vi "e1039_Magnet_PS_Control.vi"(10 "Comms Layer":T1=enum."ISOBus - RS-232", 11 "Serial Port":refnum<visa-resource-name>="COM6") -> (3 "Output Current (A)":dbl format="%.2g")   [LabVIEW 2019]
uses:
  Mercury iXX Modules/Public/Controls/Comms Transport Layer.ctl
  Mercury iXX Modules/Public/Controls/ISOBus Address.ctl
  Mercury iXX Modules/Public/Controls/Serial Settings.ctl
  Mercury iXX Modules/Public/Libraries/Magnet/Controls/Switch Heater.ctl
  Mercury iXX Modules/Public/Libraries/Magnet/Controls/PSU Actions.ctl
  Mercury iXX Modules/Public/Libraries/System/Open/Open System.vi
  Mercury iXX Modules/Public/Libraries/System/Read/Catalogue (Read).vi
  Global 2.vi
  Mercury iXX Modules/Public/Libraries/Magnet/Open/Open Magnet Device.vi
  Mercury iXX Modules/Public/Libraries/Magnet/Signals/Read/Persistant Current (Read).vi
  Mercury iXX Modules/Public/Libraries/Magnet/Signals/Read/Current (Read).vi
  Mercury iXX Modules/Public/Libraries/Magnet/Signals/Read/Voltage (Read).vi
  Mercury iXX Modules/Public/Libraries/Magnet/Signals/Read/Switch Heater Status (Read).vi
  Mercury iXX Modules/Public/Libraries/Magnet/Signals/Set/Switch Heater No Check (Set).vi
  Mercury iXX Modules/Public/Libraries/Magnet/Configuration/Set/PSU Action Status (Set).vi
  Mercury iXX Modules/Public/Libraries/Magnet/Signals/Set/Target Current (Set).vi
  Mercury iXX Modules/Public/Libraries/Magnet/Signals/Set/Target Current Rate (Set).vi
  Mercury iXX Modules/Public/Libraries/Magnet/Configuration/Read/PSU Action Status (Read).vi
  Mercury iXX Modules/Public/Libraries/Level Meter/Signals/Read/Probe Level Helium (Read).vi
  Mercury iXX Modules/Public/Libraries/Level Meter/Signals/Read/Probe Level Nitrogen (Read).vi
  Mercury iXX Modules/Mercury iXX.lvlib
  Mercury iXX Modules/Public/Libraries/Magnet.lvlib
  Mercury iXX Modules/Public/Libraries/System.lvlib
  Mercury iXX Modules/Public/Libraries/Level Meter.lvlib
panel:
  in  "Stop Button":bool
  out "Shim Relay Message":string
  out "Shim Relay Status":bool
  in  "Shim Relay SN":string="AB0NXJH7"
  out "Shim2Light":bool
  in  "Shim 2":bool
  out "Shim1Light":bool
  in  "Shim 1":bool
  in  "OK Button":bool
  in  "x":dbl=14.889566783098592 format="%#_13g"
  in  "Current NMR Central Frequency:":dbl
  in  "y":dbl=20.0
  out "SAFETY TIMEOUT":u8(slide) scale=0.0..60.0
  in  "safemode":bool=TRUE
  out "Numeric":dbl
  in  "Help Button":bool
  out "help":string="To ramp the current above 74.8 A, or faster than 2 A/min (for I<40A), 1 A/min (for 40A<I<63A) or 0.5 A/min (for I>63A), please enter the correct password.\n\nBaseline Mode: Toggle on to ramp the magnet to 1 A below the set point for the purposes of taking a baseline. Toggle off to ramp back to the set point. If the switch heater is off, it will be turned on when this button is pressed.\n\nSafety Mode: While toggled on, switch heater will automatically turn off after 20 minutes of inactivity. Enter password to change timeout duration."
  in  "Special Functions":bool
  out "Baselinetext":string
  in  "Target Species:":dbl(ring)=42.576 items=["Proton"=42.576, "Deuteron"=6.536]
  out "Heater Status 2":u8(slide) scale=0.0..60.0
  in  "Baseline Mode":bool
  out "Heater Status":u8(slide) scale=0.0..60.0
  out "String":string
  in  "Target Frequency (MHz):":dbl max=213.8870019787944
  in  "Target Field (T):":dbl max=5.02365186909983 format="%#_5g"
  in  "Axis Group":string(combo)="GRPZ"
  in  "Target Current":dbl max=74.8 format="%#_5g"
  out "concatenated string 2":string
  out "Nitrogen Fill Level":dbl(slide) scale=0.0..100.0
  out "concatenated string":string
  out "Helium Fill Level":dbl(slide) scale=0.0..100.0
  in  "stop":bool
  in  "controlslock":bool
  out "Zerolight":bool
  out "Setlight":bool
  out "Holdlight":bool
  out "Persistent Current (A)":dbl format="%.2g"
  in  "PASSWORD:":string
  out "Heater Indicator 3":bool
  in  "Switch Heater":bool
  in  "Ramp Rate (A/min)":dbl=0.5 min=0.0 max=2.0 format="%_6g"
  out "Target Current (A):":cluster{dbl, dbl}(knob)={0.0, 68.56622626412835} scale=0.0..120.0 scale format="%#_5g"
  in  "To Zero":bool
  in  "To Set":bool
  in  "Hold":bool
  out "Waveform Chart":cluster{"[0]":dbl, "[1]":dbl}(graph)
  out "Output Voltage (V)":dbl format="%.3g"
  out "Connected?":bool
  out "String 2":string
  # "Fermilab e1039 Magnet Control"
  # "For Drift Calibration:"
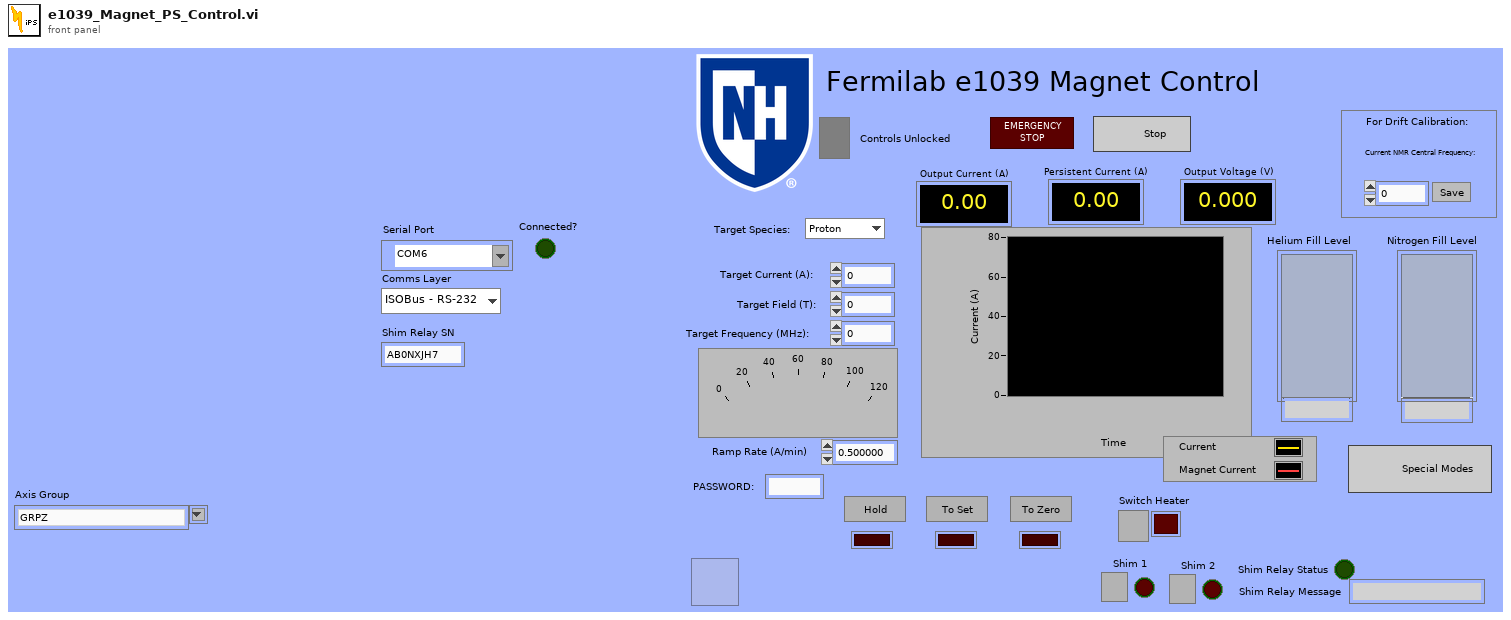
[diagram p1: front panel]
types:
  T1 = typedef "Mercury iXX.lvlib/Comms Transport Layer.ctl" = enum16{"Ethernet TCP/IP", "USB", "ISOBus - RS-232", "GPIB"}
  T2 = typedef "Mercury iXX.lvlib/Serial Settings.ctl" = cluster{"Baud Rate":u32, "Parity":u16, "Data Bits":u16, "Stop Bits":u16, "Flow Control":u16}
  T3 = typedef "Mercury iXX.lvlib/ISOBus Address.ctl" = i32
  T4 = typedef "Mercury iXX.lvlib/Mercury Reference.ctl" = cluster{"Comms":refnum<visa-resource-name>, "Device ID":string[], "Comms Layer":T1, "Command":string, "Query reference":T5}
  T5 = typedef "Mercury iXX.lvlib/Query Dynamic Reference.ctl" = refnum<vi>
  T6 = enum8{"Enabled", "Disabled", "Disabled and Grayed Out"}
  T7 = typedef "Mercury iXX.lvlib/Magnet.lvlib/PSU Actions.ctl" = string
  T8 = typedef "Mercury iXX.lvlib/Magnet.lvlib/Switch Heater.ctl" = string
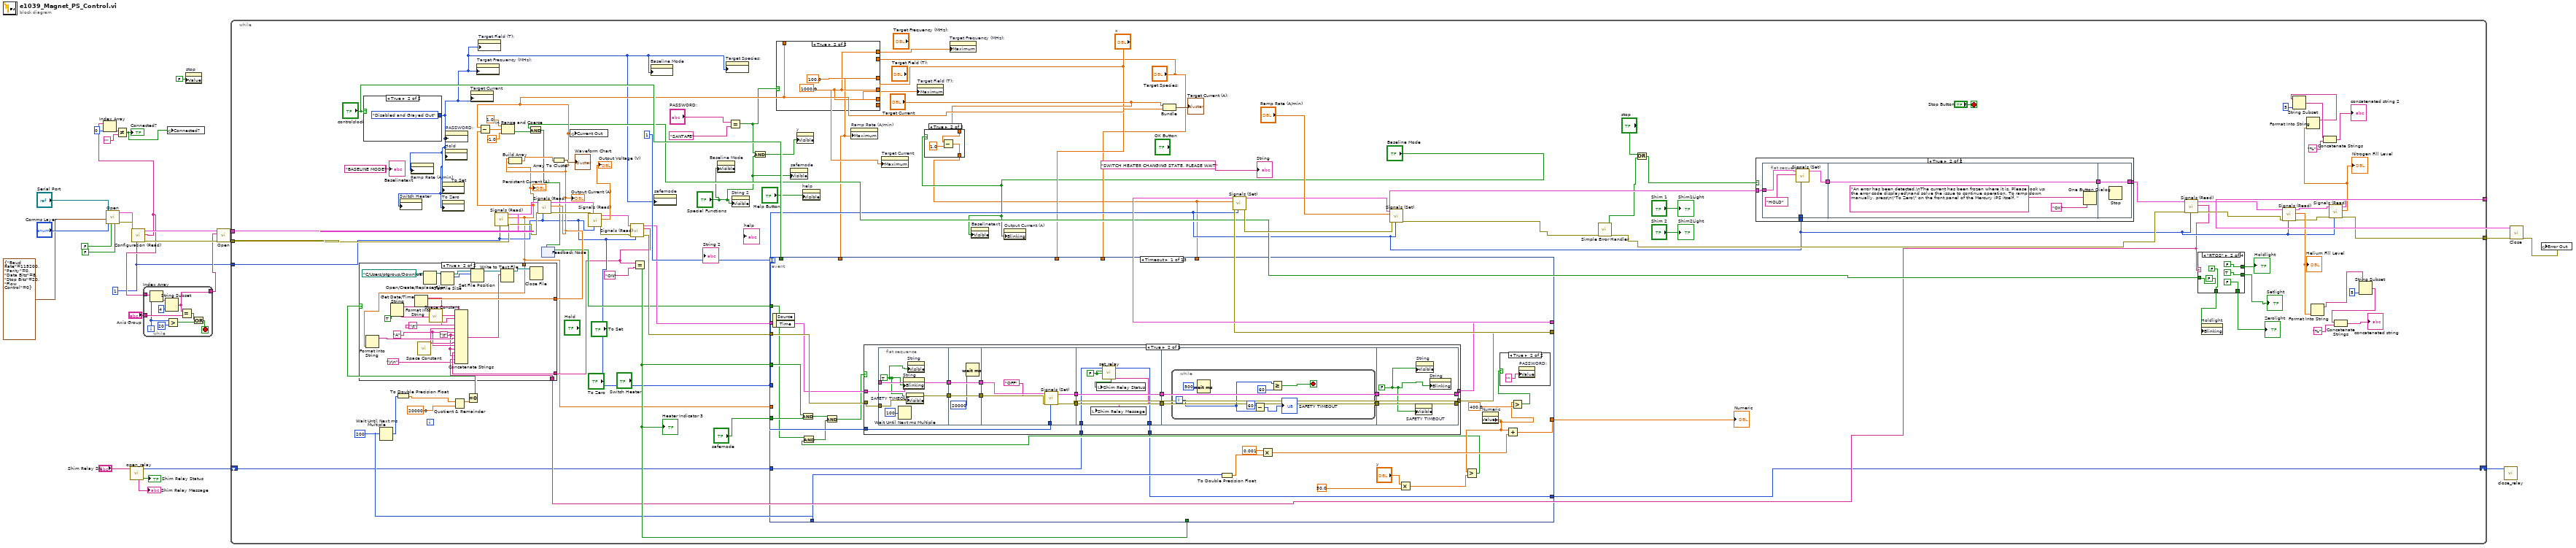
[diagram p0: block diagram]
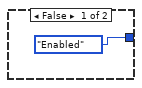
[diagram p3: hidden frame]
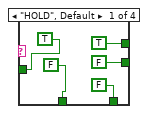
[diagram p4: hidden frame]
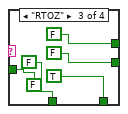
[diagram p5: hidden frame]
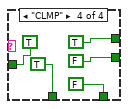
[diagram p6: hidden frame]
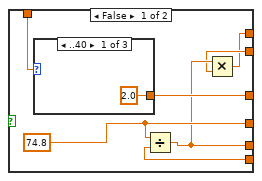
[diagram p9: hidden frame]
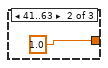
[diagram p10: hidden frame]
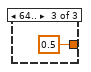
[diagram p11: hidden frame]
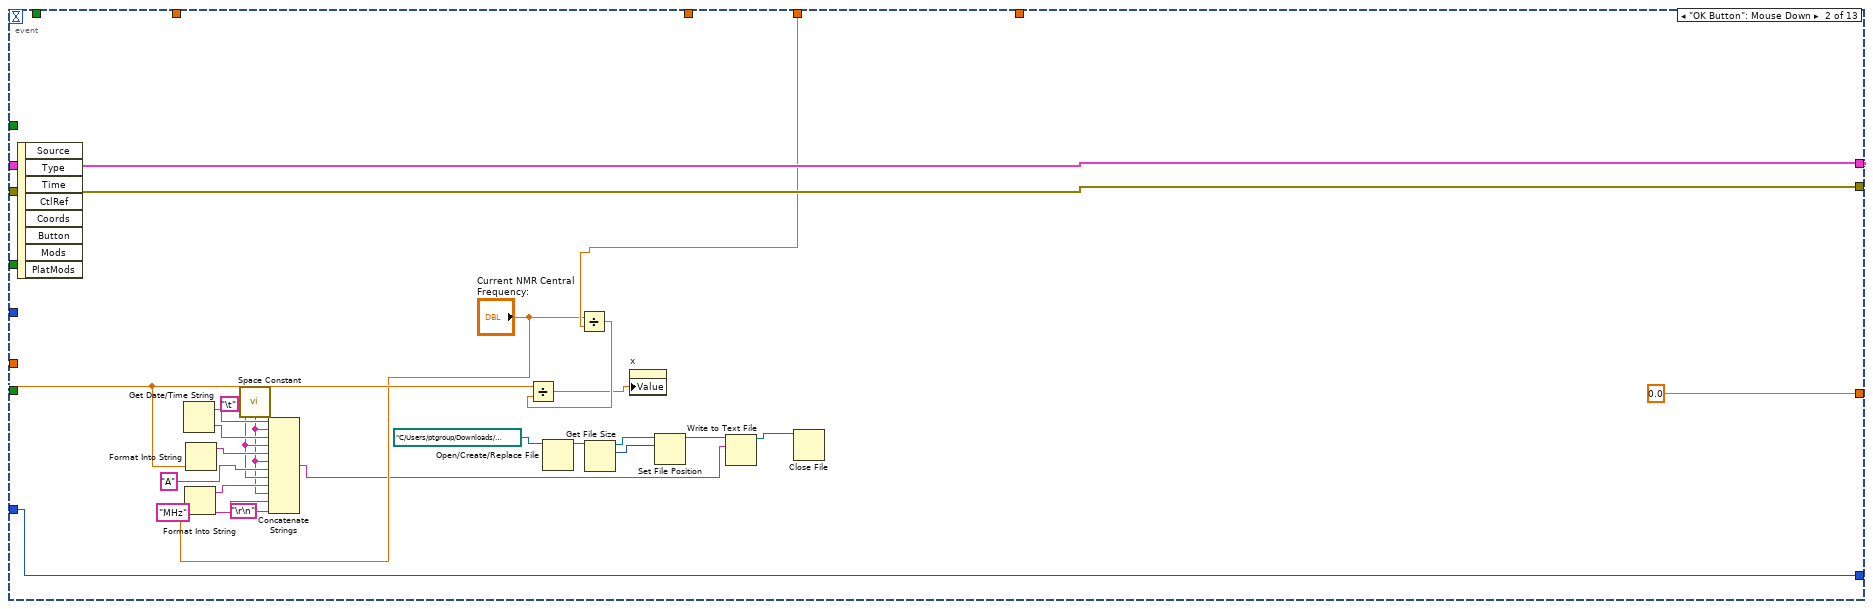
[diagram p14: hidden frame]
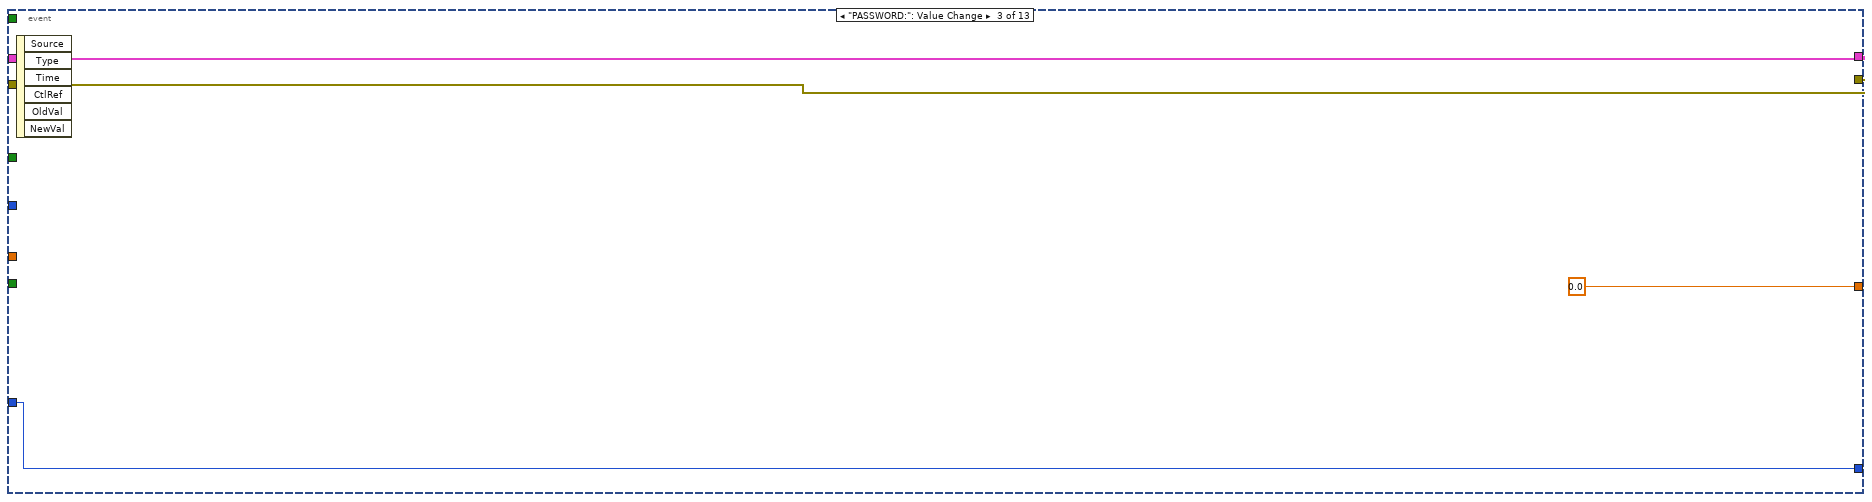
[diagram p15: hidden frame]
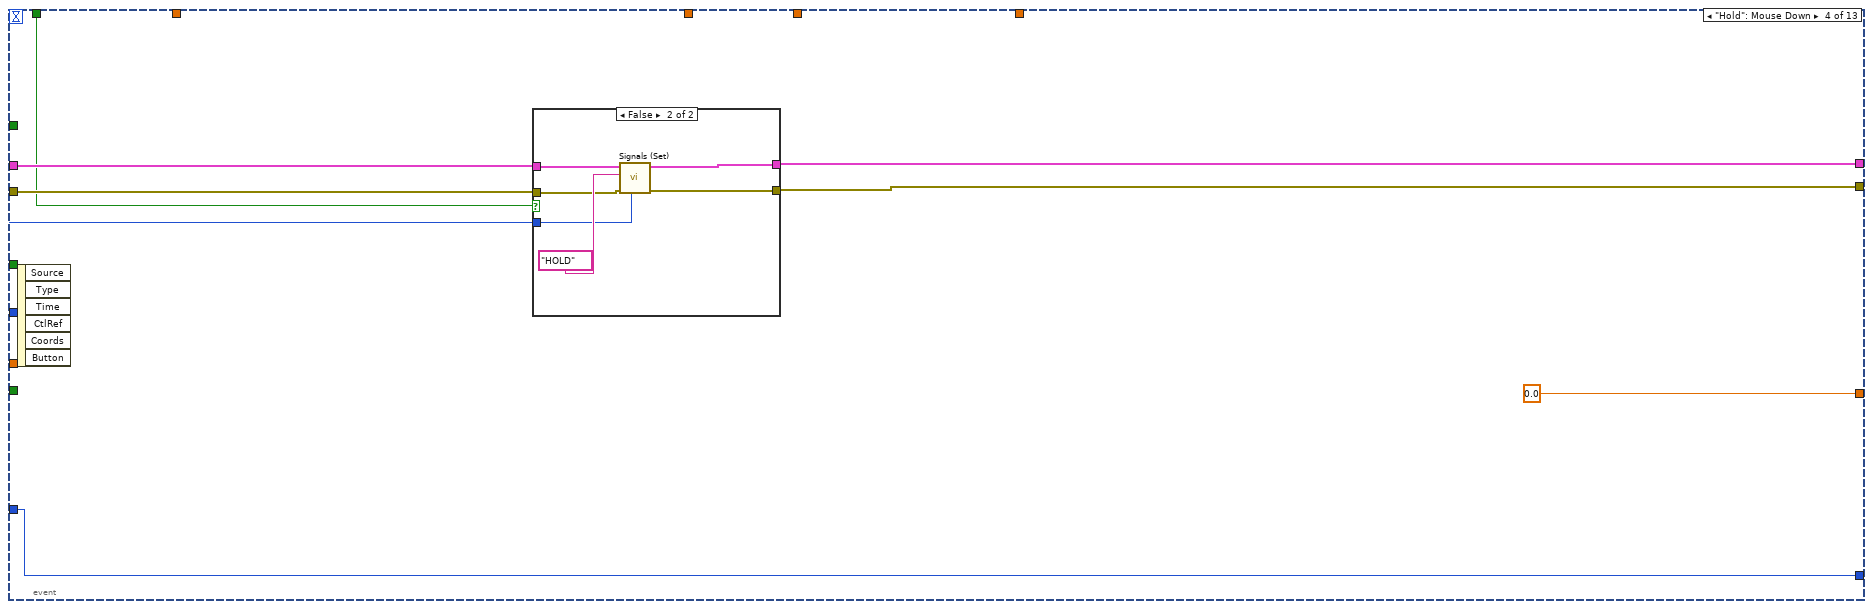
[diagram p16: hidden frame]
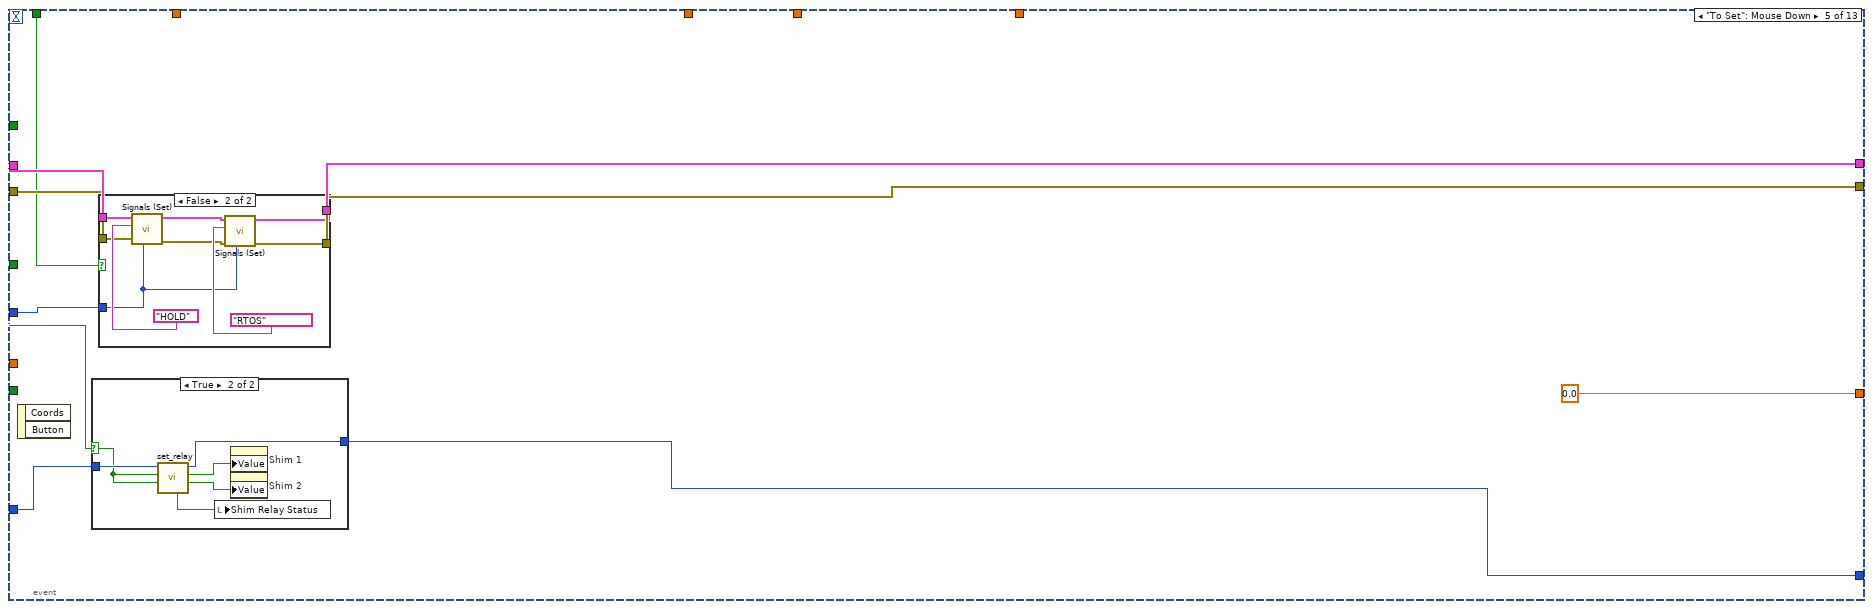
[diagram p18: hidden frame]
diagram:
  w7 = T3 1 ("ISOBUS address")
  n1 = call-poly "Open.vi"("Clear Previous Connections (False)"=FALSE, "ID Query (True)"=FALSE, "Serial Configuration"=T2 {"Baud Rate"=115200, "Parity"=0, "Data Bits"=8, "Stop Bits"=20, "Flow Control"=0}, "Comms Layer"="Comms Layer", "VISA resource name"="Serial Port") -> ("error out"=w21:errorcluster, "Mercury Reference Out"=w27:T4)  [unwired: 2 in, 3 out]
  n2 = call "open_relay.vi"("serial_number"="Shim Relay SN") -> ("status"=→"Shim Relay Status":bool, "Handle"=w2:u64, "message"=→"Shim Relay Message":string)  [unwired: 7 in, 1 out]
  n3 = call-poly "Configuration (Read).vi"("ISOBUS address"=w7, "error in"=w21, "Mercury Reference In"=w27) -> ("error out"=w20:errorcluster, "Devices"=w9:string[], "Mercury Reference Out"=w23:T4)  [unwired: 5 in, 1 out]
  n4 = Index Array(array=w9, index=0) -> (element=w24:string)
  n5 = Not Equal?(x=w24, y="") -> (x != y?=w6:bool)
  "Connected?" <- w6
  n6 = while {
    tunnel: w9 -> [w38]
    tunnel: [w29] -> w8
    tunnel: "Axis Group" -> [w35]
    i -> [w33]
    stop <- w32 stop-if-true
    n7 = Index Array(array=w38, index=w33) -> (element=w36:string)
    n8 = String Subset(string=w36, length (rest)=4 ("length (rest)")) -> (substring=w29:string)  [unwired: 1 out]
    n9 = Greater?(x=w33, y=20) -> (0:w31:bool)
    n10 = Equal?(x=w29, y=w35) -> (x = y?=w30:bool)
    n11 = Or(x=w30, y=w31) -> (x .or. y?=w32:bool)
  }
  n12 = global write "Global 2.vi" "Connected?"(w6) -> ()
  n13 = property on="stop" class="Bool (strict)"("Value"=FALSE ("stop")) -> ()  [unwired: 2 in, 2 out]
  n14 = call-poly "Open.vi"("error in (no error)"=w20, "Device Identifier"=w8, "Mercury Reference In"=w23) -> ("error out"=w19:errorcluster, "Mercury Reference Out"=w22:T4)  [unwired: 7 in]
  n15 = while {
    tunnel: w22 -> [w113]
    tunnel: w19 -> [w115]
    tunnel: [w86] -> w17
    tunnel: [w85] -> w16
    tunnel: w7 -> [w65]
    shift-right: [w40] -> w1
    shift-left: w2 -> [w41]
    stop <- "Stop Button" stop-if-true
    (unwired) "BASELINE MODE" ("Baselinetext")
    w51 = u32 200 ("millisecond multiple")
    n16 = case shown="True" "controlslock" {
      tunnel: [T6."Enabled" ("Disabled") T6."Disabled and Grayed Out" ("Disabled")] -> w45
      frame False {
      }
      frame True {
      }
    }
    n17 = Wait Until Next ms Multiple(millisecond multiple=w51) -> (millisecond timer value=w110:u32)
    n18 = To Double Precision Float(number=w110) -> (double precision float=w107:dbl)
    n19 = property on="Switch Heater" class="Bool (strict)"("DisabledEnum"=w45) -> ()  [unwired: 2 in, 2 out]
    n20 = property on="Ramp Rate (A/min)" class="DigNum (strict)"("DisabledEnum"=w45) -> ()  [unwired: 2 in, 2 out]
    n21 = property on="To Set" class="Bool"("DisabledEnum"=w45) -> ()  [unwired: 2 in, 2 out]
    n22 = property on="To Zero" class="Bool"("DisabledEnum"=w45) -> ()  [unwired: 2 in, 2 out]
    n23 = property on="Hold" class="Bool"("DisabledEnum"=w45) -> ()  [unwired: 2 in, 2 out]
    n24 = property on="PASSWORD:" class="Str"("DisabledEnum"=w45) -> ()  [unwired: 2 in, 2 out]
    n25 = Quotient & Remainder(x=w107, y=20000.0) -> (x-y*floor(x/y)=w108:dbl)  [unwired: 1 out]
    n26 = Equal To 0?(x=w108) -> (x = 0?=w109:bool)
    n27 = property on="Target Current" class="DigNum (strict)"("DisabledEnum"=w45) -> ()  [unwired: 2 in, 2 out]
    n28 = property on="Target Frequency (MHz):" class="DigNum (strict)"("DisabledEnum"=w45) -> ()  [unwired: 2 in, 2 out]
    n29 = property on="Target Field (T):" class="DigNum (strict)"("DisabledEnum"=w45) -> ()  [unwired: 2 in, 2 out]
    n30 = call-poly "Signals (Read).vi"("ISOBUS address"=w65, "error in"=w115, "Mercury Reference In"=w113) -> ("error out"=w114:errorcluster, "Persistant Current"=w46:dbl, "Mercury Reference Out"=w112:T4)  [unwired: 4 in, 2 out]
    "Persistent Current (A)" <- w46
    n31 = call-poly "Signals (Read).vi"("ISOBUS address"=w65, "error in"=w114, "Mercury Reference In"=w112) -> ("error out"=w124:errorcluster, "Current"=w72:dbl, "Mercury Reference Out"=w133:T4)  [unwired: 4 in, 2 out]
    "Output Current (A)" <- w72
    n32 = Subtract(x=w72, y=w46) -> (x-y=w106:dbl)
    n33 = In Range and Coerce(upper limit=1.0, x=w106, lower limit=-1.0) -> (In Range?=w69:bool)  [unwired: 1 out]
    n34 = Build Array(w72, w46) -> (w80:dbl[])
    n35 = feedback #1() -> (w66:bool)  [unwired: 1 in]
    n36 = Array To Cluster(array=w80) -> (cluster=→"Waveform Chart":cluster{"[0]":dbl, "[1]":dbl})
    n37 = global write "Global 2.vi" "Current Out"(w72) -> ()
    n38 = call-poly "Signals (Read).vi"("ISOBUS address"=w65, "error in"=w124, "Mercury Reference In"=w133) -> ("error out"=w123:errorcluster, "Voltage"=→"Output Voltage (V)":dbl, "Mercury Reference Out"=w127:T4)  [unwired: 4 in, 2 out]
    n39 = call-poly "Signals (Read).vi"("ISOBUS address"=w65, "error in"=w123, "Mercury Reference In"=w127) -> ("error out"=w121:errorcluster, "Switch Heater Status"=w56:string, "Mercury Reference Out"=w126:T4)  [unwired: 5 in, 1 out]
    n40 = Equal?(x=w56, y="ON") -> (x = y?=w97:bool)
    "Heater Indicator 3" <- w97
    n41 = property on="Baseline Mode" class="Bool (strict)"("DisabledEnum"=w45) -> ()  [unwired: 2 in, 2 out]
    n42 = property on="safemode" class="Bool (strict)"("DisabledEnum"=w45) -> ()  [unwired: 2 in, 2 out]
    n43 = property on="Baseline Mode" class="Bool (strict)"("Visible"="Special Functions") -> ()  [unwired: 2 in, 2 out]
    n44 = property on="Target Species:" class="Ring (strict)"("DisabledEnum"=w45) -> ()  [unwired: 2 in, 2 out]
    n45 = Equal?(x="PASSWORD:", y="SANTAFE") -> (x = y?=w49:bool)
    n46 = property on="String 2" class="Str"("Visible"="Special Functions") -> ()  [unwired: 2 in, 2 out]
    n47 = And(x=w49, y="Special Functions") -> (x .and. y?=w48:bool)
    n48 = case shown="True" w49 {
      tunnel: [w199 w206] -> w70
      tunnel: [w202 100.0 ("Data Entry Limits:Maximum")] -> w44
      tunnel: w72 -> [w201 _]
      tunnel: "x" -> [w200 _]
      tunnel: [w198 w206] -> w61
      tunnel: "Target Species:" -> [w197 _]
      tunnel: [w196 w206] -> w59
      frame False {
        w199 = 74.8 ("Data Entry Limits:Maximum")
        n49 = case shown="..40" w201 {
          tunnel: [2.0 ("Data Entry Limits:Maximum") 1.0 ("Data Entry Limits:Maximum") 0.5 ("Data Entry Limits:Maximum")] -> w202
          frame ..40 {
          }
          frame 41..63 {
          }
          frame 64.. {
          }
        }
        n50 = Divide(x=w199, y=w200) -> (x/y=w198:dbl)
        n51 = Multiply(x=w198, y=w197) -> (x*y=w196:dbl)
      }
      frame True {
        w206 = 1000.0 ("Data Entry Limits:Maximum")
      }
    }
    n52 = property on="safemode" class="Bool (strict)"("Visible"="Special Functions") -> ()  [unwired: 2 in, 2 out]
    n53 = property on="y" class="DigNum (strict)"("Visible"=w48) -> ()  [unwired: 2 in, 2 out]
    n54 = property on="help" class="Str"("Visible"="Help Button") -> ()  [unwired: 2 in, 2 out]
    n55 = property on="Ramp Rate (A/min)" class="DigNum (strict)"("Maximum"=w44) -> ()  [unwired: 2 in, 2 out]
    n56 = property on="Target Current" class="DigNum (strict)"("Maximum"=w70) -> ()  [unwired: 2 in, 2 out]
    n57 = property on="Target Field (T):" class="DigNum (strict)"("Maximum"=w61) -> ()  [unwired: 2 in, 2 out]
    n58 = case shown="True" "Baseline Mode" {
      tunnel: "Target Current" -> [w134 w136]
      tunnel: [w134 w135] -> w53
      frame False {
      }
      frame True {
        n59 = Subtract(x=w136, y=1.0) -> (x-y=w135:dbl)
      }
    }
    n60 = event shown="[0] Timeout" {
      selector: _ -> [_ _ _ _ _ _ _ _ _ _ _ _ _]
      dyn-events: _ -> [_ _ _ _ _ _ _ _ _ _ _ _ _]
      timeout: 1 -> [_ _ _ _ _ _ _ _ _ _ _ _ _]
      tunnel: [w222 w308 w313 w320 w339 w366 w392 w486 w577 w588 w598 w602 w611] -> w129
      tunnel: w126 -> [w223 w308 w313 w321 w338 w367 w393 w490 w577 w588 w598 w602 w611]
      tunnel: w97 -> [w219 _ _ _ w332 w360 w394 w492 _ _ _ _ _]
      tunnel: w121 -> [w224 w309 w312 w319 w337 w365 w391 w488 w576 w587 w597 w601 w610]
      tunnel: [w221 w309 w312 w318 w336 w364 w390 w487 w576 w587 w597 w601 w610] -> w120
      tunnel: w66 -> [w210 _ _ _ _ _ w389 w489 _ _ _ _ _]
      tunnel: w97 -> [_ _ _ _ _ _ w388 _ _ _ _ _ _]
      tunnel: "controlslock" -> [_ _ _ w317 w335 w363 w387 _ _ _ _ _ _]
      tunnel: w65 -> [w225 _ _ w316 w334 w362 w386 w485 _ _ _ _ _]
      tunnel: "x" -> [_ _ _ _ _ _ _ _ _ _ w595 w607 w613]
      tunnel: "Target Species:" -> [_ w306 _ _ _ _ _ _ _ _ w593 w605 w615]
      tunnel: w53 -> [_ _ _ _ _ _ _ w480 _ _ _ _ _]
      tunnel: [w228 0.0 0.0 0.0 0.0 0.0 0.0 0.0 0.0 0.0 0.0 0.0 0.0] -> w52
      tunnel: w51 -> [w232 _ _ _ _ _ _ _ _ _ _ _ _]
      tunnel: "safemode" -> [w220 _ _ _ _ _ _ _ _ _ _ _ _]
      tunnel: w46 -> [_ w295 _ _ _ _ _ _ _ _ _ _ _]
      tunnel: w44 -> [_ _ _ _ _ _ _ w479 _ _ _ _ _]
      tunnel: w41 -> [w209 w285 w310 w314 w331 w359 w384 w472 w573 w584 w590 w599 w608]
      tunnel: [w208 w285 w310 w314 w330 w358 w383 w471 w572 w583 w590 w599 w608] -> w40
      event Timeout {
        n61 = event-data() -> ()  [unwired: 1 in, 2 out]
        n62 = And(x=w219, y=w220) -> (x .and. y?=w211:bool)
        n63 = To Double Precision Float(number=w232) -> (double precision float=w231:dbl)
        n64 = Multiply(x=0.001, y=w231) -> (x*y=w229:dbl)
        n65 = Multiply(x="y", y=50.0) -> (x*y=w214:dbl)
        n66 = property on="Numeric" class="DigNum (strict)"() -> ("Value"=w218:dbl)  [unwired: 2 in, 2 out]
        n67 = Greater?(x=w218, y=w214) -> (0:w217:bool)
        n68 = And(x=w210, y=w217) -> (x .and. y?=w212:bool)
        n69 = And(x=w211, y=w212) -> (x .and. y?=w213:bool)
        n70 = case shown="True" w213 {
          tunnel: w223 -> [w235 w249]
          tunnel: [w235 w252] -> w222
          tunnel: w224 -> [w234 w251]
          tunnel: [w234 w250] -> w221
          tunnel: w225 -> [_ w248]
          tunnel: w209 -> [w233 w237]
          tunnel: [w233 w236] -> w208
          frame False {
          }
          frame True {
            n71 = flat-sequence {
              tunnel: [w256] -> w245
              tunnel: w249 -> [w256]
              tunnel: [w254] -> w243
              tunnel: w251 -> [w254]
              tunnel: w245 -> [w259]
              tunnel: [w259] -> w244
              tunnel: w243 -> [w258]
              tunnel: [w258] -> w242
              tunnel: w244 -> [w265]
              tunnel: w242 -> [w263]
              tunnel: [w264] -> w241
              tunnel: [w262] -> w239
              tunnel: w248 -> [w261]
              tunnel: w241 -> [w272]
              tunnel: [w272] -> w240
              tunnel: w239 -> [w271]
              tunnel: [w271] -> w238
              tunnel: w237 -> [w270]
              tunnel: [w268] -> w236
              tunnel: w240 -> [w274]
              tunnel: w238 -> [w273]
              tunnel: [w274] -> w247
              tunnel: [w273] -> w246
              tunnel: [w282] -> w250
              tunnel: [w283] -> w252
              tunnel: w247 -> [w283]
              tunnel: w246 -> [w282]
              frame #0 {
                w253 = TRUE ("Visible")
                n72 = Wait Until Next ms Multiple(millisecond multiple=u32 100) -> ()  [unwired: 1 out]
                n73 = property on="String" class="Str"("Blinking"=w253) -> ()  [unwired: 2 in, 2 out]
                n74 = property on="SAFETY TIMEOUT" class="Slide (strict)"("Visible"=w253) -> ()  [unwired: 2 in, 2 out]
                n75 = property on="String" class="Str"("Visible"=w253) -> ()  [unwired: 2 in, 2 out]
              }
              frame #1 {
                n76 = Wait (ms)(milliseconds to wait=u32 20000) -> ()  [unwired: 1 out]
              }
              frame #2 {
                n77 = call-poly "Signals (Set).vi"("ISOBUS address"=w261, "error in"=w263, "Set Switch Heater"=T8 "OFF", "Mercury Reference In"=w265) -> ("error out"=w262:errorcluster, "Mercury Reference Out"=w264:T4)  [unwired: 4 in, 2 out]
              }
              frame #3 {
                w269 = FALSE ("ch_1")
                n78 = call "set_relay.vi"("ch_2"=w269, "ch_1"=w269, "Handle"=w270) -> ("message"=w266:string, "Handle_out"=w268:u64, "status"=w267:bool)  [unwired: 4 in, 2 out]
                n79 = local write "Shim Relay Message"(w266) -> ()
                n80 = local write "Shim Relay Status"(w267) -> ()
              }
              frame #4 {
                n81 = while {
                  i -> [w277]
                  stop <- w279 stop-if-true
                  n82 = Wait (ms)(milliseconds to wait=u32 500) -> ()  [unwired: 1 out]
                  n83 = Subtract(x=60, y=w277) -> (x-y=→"SAFETY TIMEOUT":i32)
                  n84 = Greater Or Equal?(x=w277, y=60) -> (x >= y?=w279:bool)
                }
              }
              frame #5 {
                w281 = FALSE ("Visible")
                n85 = property on="SAFETY TIMEOUT" class="Slide (strict)"("Visible"=w281) -> ()  [unwired: 2 in, 2 out]
                n86 = property on="String" class="Str"("Visible"=w281) -> ()  [unwired: 2 in, 2 out]
                n87 = property on="String" class="Str"("Blinking"=w281) -> ()  [unwired: 2 in, 2 out]
              }
            }
          }
        }
        n88 = Add(x=w218, y=w229) -> (x+y=w228:dbl)
        n89 = Greater?(x=w218, y=400.0) -> (0:w226:bool)
        n90 = case shown="True" w226 {
          frame False {
          }
          frame True {
            n91 = property on="PASSWORD:" class="Str"("Value"="" ("PASSWORD:")) -> ()  [unwired: 2 in, 2 out]
          }
        }
      }
      event "OK Button": Mouse Down {
        w292 = "\t"
        n92 = event-data() -> ()  [unwired: 1 in, 8 out]
        n93 = Get Date/Time String() -> (date string=w297:string, time string=w296:string)  [unwired: 3 in]
        n94 = Format Into String("Current NMR Central Frequency:") -> (resulting string=w290:string)  [unwired: 3 in, 1 out]
        n95 = Format Into String(w295) -> (resulting string=w294:string)  [unwired: 3 in, 1 out]
        n96 = call <vilib>:"Space Constant.vi"() -> ("String"=w289:string)
        n97 = Concatenate Strings(w297, w289, w296, w292, w294, w289, "A", w292, w290, w289, "MHz", "\r\n") -> (w286:string)
        n98 = Open/Create/Replace File(file path (use dialog)=path "C:/Users/ptgroup/Downloads/ipsControl2013 new Folder/ipsControl2013 new Folder/C/Users/poltarg/Documents/currentcal.txt" ("file (use dialog)")) -> (refnum out=w302:refnum<file>)  [unwired: 5 in, 2 out]
        n99 = Divide(x="Current NMR Central Frequency:", y=w306) -> (x/y=w305:dbl)
        n100 = Divide(x=w295, y=w305) -> (x/y=w304:dbl)
        n101 = Get File Size(file=w302) -> (refnum out=w301:refnum<file>, size (in bytes)=w300:i64)  [unwired: 1 in, 1 out]
        n102 = property on="x" class="DigNum (strict)"("Value"=w304) -> ()  [unwired: 2 in, 2 out]
        n103 = Set File Position(offset (in bytes) (0)=w300, refnum=w301) -> (refnum out=w299:refnum<file>)  [unwired: 2 in, 1 out]
        n104 = Write to Text File(file (use dialog)=w299, text=w286) -> (refnum out=w298:refnum<file>)  [unwired: 2 in, 2 out]
        n105 = Close File(refnum=w298) -> ()  [unwired: 1 in, 2 out]
      }
      event "PASSWORD:": Value Change {
        n106 = event-data() -> ()  [unwired: 1 in, 6 out]
      }
      event "Hold": Mouse Down {
        n107 = event-data() -> ()  [unwired: 1 in, 6 out]
        n108 = case shown="False" w317 {
          tunnel: w321 -> [w323 w328]
          tunnel: [w323 w327] -> w320
          tunnel: w319 -> [w322 w326]
          tunnel: [w322 w325] -> w318
          tunnel: w316 -> [_ w324]
          frame True {
          }
          frame False {
            n109 = call-poly "Signals (Set).vi"("ISOBUS address"=w324, "error in"=w326, "PSU Act Stat"=T7 "HOLD", "Mercury Reference In"=w328) -> ("error out"=w325:errorcluster, "Mercury Reference Out"=w327:T4)  [unwired: 4 in, 2 out]
          }
        }
      }
      event "To Set": Mouse Down {
        n110 = event-data() -> ()  [unwired: 1 in, 2 out]
        n111 = case shown="True" w332 {
          selector: w332 -> [_ w343]
          tunnel: w331 -> [w340 w346]
          tunnel: [w340 w342] -> w330
          frame False {
          }
          frame True {
            n112 = call "set_relay.vi"("ch_2"=w343, "ch_1"=w343, "Handle"=w346) -> ("ch_2_out"=w345:bool, "ch_1_out"=w344:bool, "Handle_out"=w342:u64, "status"=w341:bool)  [unwired: 4 in, 1 out]
            n113 = local write "Shim Relay Status"(w341) -> ()
            n114 = property on="Shim 1" class="Bool (strict)"("Value"=w344) -> ()  [unwired: 2 in, 2 out]
            n115 = property on="Shim 2" class="Bool (strict)"("Value"=w345) -> ()  [unwired: 2 in, 2 out]
          }
        }
        n116 = case shown="False" w335 {
          tunnel: [w348 w356] -> w339
          tunnel: w338 -> [w348 w353]
          tunnel: w337 -> [w347 w352]
          tunnel: [w347 w350] -> w336
          tunnel: w334 -> [_ w349]
          frame True {
          }
          frame False {
            n117 = call-poly "Signals (Set).vi"("ISOBUS address"=w349, "error in"=w352, "PSU Act Stat"=T7 "HOLD", "Mercury Reference In"=w353) -> ("error out"=w351:errorcluster, "Mercury Reference Out"=w354:T4)  [unwired: 4 in, 2 out]
            n118 = call-poly "Signals (Set).vi"("ISOBUS address"=w349, "error in"=w351, "PSU Act Stat"=T7 "RTOS", "Mercury Reference In"=w354) -> ("error out"=w350:errorcluster, "Mercury Reference Out"=w356:T4)  [unwired: 4 in, 2 out]
          }
        }
      }
      event "To Zero": Mouse Down {
        n119 = event-data() -> ()  [unwired: 1 in, 8 out]
        n120 = case shown="True" w360 {
          selector: w360 -> [_ w373]
          tunnel: w359 -> [w368 w374]
          tunnel: [w368 w370] -> w358
          frame False {
          }
          frame True {
            n121 = call "set_relay.vi"("ch_2"=w373, "ch_1"=w373, "Handle"=w374) -> ("ch_2_out"=w371:bool, "ch_1_out"=w372:bool, "Handle_out"=w370:u64, "status"=w369:bool)  [unwired: 4 in, 1 out]
            n122 = local write "Shim Relay Status"(w369) -> ()
            n123 = property on="Shim 1" class="Bool (strict)"("Value"=w372) -> ()  [unwired: 2 in, 2 out]
            n124 = property on="Shim 2" class="Bool (strict)"("Value"=w371) -> ()  [unwired: 2 in, 2 out]
          }
        }
        n125 = case shown="False" w363 {
          tunnel: w367 -> [w376 w381]
          tunnel: [w376 w380] -> w366
          tunnel: w365 -> [w375 w379]
          tunnel: [w375 w378] -> w364
          tunnel: w362 -> [_ w377]
          frame True {
          }
          frame False {
            n126 = call-poly "Signals (Set).vi"("ISOBUS address"=w377, "error in"=w379, "PSU Act Stat"=T7 "RTOZ", "Mercury Reference In"=w381) -> ("error out"=w378:errorcluster, "Mercury Reference Out"=w380:T4)  [unwired: 4 in, 2 out]
          }
        }
      }
      event "Switch Heater": Mouse Down {
        n127 = event-data() -> ()  [unwired: 1 in, 1 out]
        n128 = case shown="False" w387 {
          tunnel: w394 -> [_ w407]
          tunnel: w393 -> [w397 w406]
          tunnel: [w397 w405] -> w392
          tunnel: w391 -> [w396 w404]
          tunnel: [w396 w403] -> w390
          tunnel: w389 -> [_ w402]
          tunnel: w388 -> [_ w401]
          tunnel: w386 -> [_ w400]
          tunnel: w384 -> [w395 w399]
          tunnel: [w395 w398] -> w383
          frame True {
          }
          frame False {
            n129 = case shown="True" w402 {
              tunnel: w407 -> [_ w428]
              tunnel: w406 -> [w412 w424]
              tunnel: [w412 w427] -> w405
              tunnel: w404 -> [w411 w426]
              tunnel: [w411 w425] -> w403
              tunnel: w401 -> [_ w423]
              tunnel: w400 -> [_ w422]
              tunnel: w399 -> [w408 w414]
              tunnel: [w408 w413] -> w398
              frame False {
                n130 = One Button Dialog(message="The output current and magnet current are more than 1 amp apart, or the iPS is ramping!\nPlease ramp until they match and set to 'Hold' before turning on the switch heater.", button name ("OK")="OK") -> ()  [unwired: 1 out]
              }
              frame True {
                n131 = flat-sequence {
                  tunnel: [w436] -> w431
                  tunnel: [w435] -> w430
                  tunnel: w428 -> [w436]
                  tunnel: w424 -> [w435]
                  tunnel: [w433] -> w429
                  tunnel: w426 -> [w433]
                  tunnel: w431 -> [w437]
                  tunnel: w430 -> [w442]
                  tunnel: w429 -> [w440]
                  tunnel: [w441] -> w419
                  tunnel: [w439] -> w417
                  tunnel: w422 -> [w438]
                  tunnel: [w437] -> w415
                  tunnel: w419 -> [w454]
                  tunnel: [w454] -> w418
                  tunnel: w417 -> [w453]
                  tunnel: [w453] -> w416
                  tunnel: w415 -> [w452]
                  tunnel: w414 -> [w451]
                  tunnel: [w447] -> w413
                  tunnel: w418 -> [w457]
                  tunnel: w416 -> [w456]
                  tunnel: w423 -> [w455]
                  tunnel: [w457] -> w421
                  tunnel: [w456] -> w420
                  tunnel: [w469] -> w425
                  tunnel: [w470] -> w427
                  tunnel: w421 -> [w470]
                  tunnel: w420 -> [w469]
                  frame #0 {
                    w432 = TRUE ("Visible")
                    n132 = property on="String" class="Str"("Blinking"=w432) -> ()  [unwired: 2 in, 2 out]
                    n133 = property on="String" class="Str"("Visible"=w432) -> ()  [unwired: 2 in, 2 out]
                    n134 = property on="Heater Status" class="Slide (strict)"("Visible"=w432) -> ()  [unwired: 2 in, 2 out]
                    n135 = Wait Until Next ms Multiple(millisecond multiple=u32 100) -> ()  [unwired: 1 out]
                  }
                  frame #1 {
                    n136 = Select(t=T8 "OFF" ("Set Switch Heater"), s=w437, f=T8 "ON" ("Set Switch Heater")) -> (s? t:f=w443:T8)
                    n137 = call-poly "Signals (Set).vi"("ISOBUS address"=w438, "error in"=w440, "Set Switch Heater"=w443, "Mercury Reference In"=w442) -> ("error out"=w439:errorcluster, "Mercury Reference Out"=w441:T4)  [unwired: 4 in, 2 out]
                  }
                  frame #2 {
                    n138 = Not(x=w452) -> (.not. x?=w450:bool)
                    n139 = call "set_relay.vi"("ch_2"=w450, "ch_1"=w450, "Handle"=w451) -> ("ch_2_out"=w448:bool, "ch_1_out"=w449:bool, "Handle_out"=w447:u64, "status"=w446:bool)  [unwired: 4 in, 1 out]
                    n140 = local write "Shim Relay Status"(w446) -> ()
                    n141 = property on="Shim 1" class="Bool (strict)"("Value"=w449) -> ()  [unwired: 2 in, 2 out]
                    n142 = property on="Shim 2" class="Bool (strict)"("Value"=w448) -> ()  [unwired: 2 in, 2 out]
                  }
                  frame #3 {
                    n143 = while {
                      tunnel: w455 -> [w458]
                      i -> [w460]
                      stop <- w462 stop-if-true
                      n144 = Wait (ms)(milliseconds to wait=u32 500) -> ()  [unwired: 1 out]
                      n145 = case shown="True" w458 {
                        tunnel: [w464 w465] -> w459
                        tunnel: w460 -> [w464 w467]
                        frame False {
                        }
                        frame True {
                          n146 = Subtract(x=60, y=w467) -> (x-y=w465:i32)
                        }
                      }
                      "Heater Status" <- w459
                      n147 = Greater Or Equal?(x=w460, y=60) -> (x >= y?=w462:bool)
                    }
                  }
                  frame #4 {
                    w468 = FALSE ("Visible")
                    n148 = property on="String" class="Str"("Blinking"=w468) -> ()  [unwired: 2 in, 2 out]
                    n149 = property on="Heater Status" class="Slide (strict)"("Visible"=w468) -> ()  [unwired: 2 in, 2 out]
                    n150 = property on="String" class="Str"("Visible"=w468) -> ()  [unwired: 2 in, 2 out]
                  }
                }
              }
            }
          }
        }
      }
      event "Baseline Mode": Mouse Down {
        n151 = Not(x=w492) -> (.not. x?=w491:bool)
        n152 = event-data() -> ()  [unwired: 1 in, 8 out]
        n153 = flat-sequence {
          tunnel: w491 -> [w499]
          tunnel: w490 -> [w498]
          tunnel: w489 -> [w497]
          tunnel: w488 -> [w496]
          tunnel: [w495] -> w483
          tunnel: [w494] -> w482
          tunnel: w485 -> [w493]
          tunnel: [w493] -> w481
          tunnel: w483 -> [w545]
          tunnel: w482 -> [w546]
          tunnel: [w544] -> w478
          tunnel: w481 -> [w547]
          tunnel: [w547] -> w476
          tunnel: w480 -> [w548]
          tunnel: [w543] -> w474
          tunnel: w479 -> [w542]
          tunnel: w478 -> [w558]
          tunnel: [w558] -> w477
          tunnel: w476 -> [w557]
          tunnel: [w557] -> w475
          tunnel: w474 -> [w556]
          tunnel: [w556] -> w473
          tunnel: w472 -> [w554]
          tunnel: [w549] -> w471
          tunnel: [w566] -> w486
          tunnel: [w564] -> w487
          tunnel: w477 -> [w560]
          tunnel: w475 -> [w561]
          tunnel: w473 -> [w559]
          frame #0 {
            n154 = case shown="True" w499 {
              tunnel: w498 -> [w500 w507]
              tunnel: w497 -> [_ w506]
              tunnel: w496 -> [w501 w505]
              tunnel: [w501 w504] -> w495
              tunnel: [w500 w503] -> w494
              tunnel: w493 -> [_ w502]
              frame False {
              }
              frame True {
                n155 = case shown="True" w506 {
                  tunnel: w507 -> [w511 w517]
                  tunnel: [w511 w522] -> w503
                  tunnel: w505 -> [w510 w515]
                  tunnel: [w510 w521] -> w504
                  tunnel: w502 -> [_ w514]
                  frame False {
                    n156 = One Button Dialog(message="The output current and magnet current are more than 1 amp apart, or the iPS is ramping!\nPlease ramp until they match and set to 'Hold' before turning on the switch heater.", button name ("OK")="OK") -> ()  [unwired: 1 out]
                  }
                  frame True {
                    n157 = flat-sequence {
                      tunnel: w517 -> [w525]
                      tunnel: [w525] -> w518
                      tunnel: [w524] -> w516
                      tunnel: w515 -> [w524]
                      tunnel: [w532] -> w513
                      tunnel: [w531] -> w512
                      tunnel: w518 -> [w529]
                      tunnel: w516 -> [w528]
                      tunnel: w514 -> [w527]
                      tunnel: w513 -> [w534]
                      tunnel: w512 -> [w533]
                      tunnel: [w534] -> w520
                      tunnel: [w533] -> w519
                      tunnel: [w540] -> w521
                      tunnel: [w541] -> w522
                      tunnel: w520 -> [w541]
                      tunnel: w519 -> [w540]
                      frame #0 {
                        w523 = TRUE ("Visible")
                        n158 = property on="Heater Status 2" class="Slide (strict)"("Visible"=w523) -> ()  [unwired: 2 in, 2 out]
                        n159 = property on="String" class="Str"("Visible"=w523) -> ()  [unwired: 2 in, 2 out]
                        n160 = Wait Until Next ms Multiple(millisecond multiple=u32 100) -> ()  [unwired: 1 out]
                        n161 = property on="String" class="Str"("Blinking"=w523) -> ()  [unwired: 2 in, 2 out]
                      }
                      frame #1 {
                        n162 = call-poly "Signals (Set).vi"("ISOBUS address"=w527, "error in"=w528, "Set Switch Heater"=T8 "ON", "Mercury Reference In"=w529) -> ("error out"=w531:errorcluster, "Mercury Reference Out"=w532:T4)  [unwired: 4 in, 2 out]
                      }
                      frame #2 {
                        n163 = while {
                          i -> [w535]
                          stop <- w537 stop-if-true
                          n164 = Wait (ms)(milliseconds to wait=u32 500) -> ()  [unwired: 1 out]
                          n165 = Greater Or Equal?(x=w535, y=60) -> (x >= y?=w537:bool)
                          "Heater Status 2" <- w535
                        }
                      }
                      frame #3 {
                        w539 = FALSE ("Visible")
                        n166 = property on="Heater Status 2" class="Slide (strict)"("Visible"=w539) -> ()  [unwired: 2 in, 2 out]
                        n167 = property on="String" class="Str"("Visible"=w539) -> ()  [unwired: 2 in, 2 out]
                        n168 = property on="String" class="Str"("Blinking"=w539) -> ()  [unwired: 2 in, 2 out]
                      }
                    }
                  }
                }
              }
            }
          }
          frame #1 {
            n169 = call-poly "Signals (Set).vi"("ISOBUS address"=w547, "error in"=w545, "Target Current"=w548, "Mercury Reference In"=w546) -> ("error out"=w543:errorcluster, "Mercury Reference Out"=w544:T4)  [unwired: 4 in, 2 out]
            n170 = property on="Ramp Rate (A/min)" class="DigNum (strict)"("Value"=w542) -> ()  [unwired: 2 in, 2 out]
          }
          frame #2 {
            w553 = TRUE
            n171 = call "set_relay.vi"("ch_2"=w553, "ch_1"=w553, "Handle"=w554) -> ("ch_2_out"=w551:bool, "ch_1_out"=w552:bool, "Handle_out"=w549:u64, "status"=w550:bool)  [unwired: 4 in, 1 out]
            n172 = Wait (ms)(milliseconds to wait=u32 4000) -> ()  [unwired: 1 out]
            n173 = local write "Shim Relay Status"(w550) -> ()
            n174 = property on="Shim 1" class="Bool (strict)"("Value"=w552) -> ()  [unwired: 2 in, 2 out]
            n175 = property on="Shim 2" class="Bool (strict)"("Value"=w551) -> ()  [unwired: 2 in, 2 out]
          }
          frame #3 {
            n176 = call-poly "Signals (Set).vi"("ISOBUS address"=w561, "error in"=w559, "PSU Act Stat"=T7 "HOLD", "Mercury Reference In"=w560) -> ("error out"=w565:errorcluster, "Mercury Reference Out"=w567:T4)  [unwired: 4 in, 2 out]
            n177 = call-poly "Signals (Set).vi"("ISOBUS address"=w561, "error in"=w565, "PSU Act Stat"=T7 "RTOS", "Mercury Reference In"=w567) -> ("error out"=w564:errorcluster, "Mercury Reference Out"=w566:T4)  [unwired: 4 in, 2 out]
          }
        }
      }
      event "Shim 1": Value Change {
        n178 = event-data() -> ("NewVal"=w574:bool)  [unwired: 1 in, 5 out]
        n179 = local read "Shim 2"() -> (w575:bool)
        n180 = call "set_relay.vi"("ch_2"=w575, "ch_1"=w574, "Handle"=w573) -> ("message"=w568:string, "ch_2_out"=w570:bool, "ch_1_out"=w571:bool, "Handle_out"=w572:u64, "status"=w569:bool)  [unwired: 4 in]
        n181 = local write "Shim Relay Status"(w569) -> ()
        n182 = local write "Shim1Light"(w571) -> ()
        n183 = local write "Shim2Light"(w570) -> ()
        n184 = local write "Shim Relay Message"(w568) -> ()
      }
      event "Shim 2": Value Change {
        n185 = event-data() -> ("NewVal"=w585:bool)  [unwired: 1 in, 5 out]
        n186 = local read "Shim 1"() -> (w586:bool)
        n187 = call "set_relay.vi"("ch_2"=w585, "ch_1"=w586, "Handle"=w584) -> ("message"=w579:string, "ch_2_out"=w582:bool, "ch_1_out"=w581:bool, "Handle_out"=w583:u64, "status"=w580:bool)  [unwired: 4 in]
        n188 = local write "Shim Relay Message"(w579) -> ()
        n189 = local write "Shim Relay Status"(w580) -> ()
        n190 = local write "Shim1Light"(w581) -> ()
        n191 = local write "Shim2Light"(w582) -> ()
      }
      event "Target Current": Value Change {
        n192 = event-data() -> ("NewVal"=w596:dbl)  [unwired: 1 in]
        n193 = Divide(x=w596, y=w595) -> (x/y=w594:dbl)
        n194 = local write "Target Field (T):"(w594) -> ()
        n195 = Multiply(x=w594, y=w593) -> (x*y=w592:dbl)
        n196 = local write "Target Frequency (MHz):"(w592) -> ()
      }
      event "Target Field (T):": Value Change {
        n197 = event-data() -> ("NewVal"=w604:dbl)  [unwired: 1 in]
        n198 = Multiply(x=w607, y=w604) -> (x*y=w606:dbl)
        n199 = Multiply(x=w605, y=w604) -> (x*y=w603:dbl)
        n200 = local write "Target Current"(w606) -> ()
        n201 = local write "Target Frequency (MHz):"(w603) -> ()
      }
      event "Target Frequency (MHz):": Value Change {
        n202 = event-data() -> ("NewVal"=w616:dbl)  [unwired: 1 in]
        n203 = Divide(x=w616, y=w615) -> (x/y=w614:dbl)
        n204 = Multiply(x=w613, y=w614) -> (x*y=w612:dbl)
        n205 = local write "Target Field (T):"(w614) -> ()
        n206 = local write "Target Current"(w612) -> ()
      }
    }
    "Numeric" <- w52
    n207 = property on="Target Frequency (MHz):" class="DigNum (strict)"("Maximum"=w59) -> ()  [unwired: 2 in, 2 out]
    n208 = property on="Baselinetext" class="Str"("Visible"="Baseline Mode") -> ()  [unwired: 2 in, 2 out]
    n209 = property on="Output Current (A)" class="DigNum (strict)"("Blinking"="Baseline Mode") -> ()  [unwired: 2 in, 2 out]
    n210 = Bundle("Target Current"="Target Current", "Current"=w72) -> (→"Target Current (A):":cluster{"Target Current":dbl, "Current":dbl})  [unwired: 1 in]
    n211 = call-poly "Signals (Set).vi"("ISOBUS address"=w65, "error in"=w120, "Target Current"=w53, "Mercury Reference In"=w129) -> ("error out"=w122:errorcluster, "Mercury Reference Out"=w128:T4)  [unwired: 4 in, 2 out]
    n212 = call-poly "Signals (Set).vi"("ISOBUS address"=w65, "error in"=w122, "Target Current Rate"="Ramp Rate (A/min)", "Mercury Reference In"=w128) -> ("error out"=w117:errorcluster, "Mercury Reference Out"=w116:T4)  [unwired: 4 in, 2 out]
    n213 = call <vilib>:"Simple Error Handler.vi"("error in (no error)"=w117) -> ("error?"=w96:bool, "error out"=w102:errorcluster)  [unwired: 4 in, 3 out]
    n214 = Or(x="stop", y=w96) -> (x .or. y?=w94:bool)
    n215 = case shown="True" w94 {
      tunnel: w116 -> [w182 w187]
      tunnel: [w182 w186] -> w103
      tunnel: w65 -> [_ w183]
      frame False {
      }
      frame True {
        n216 = flat-sequence {
          tunnel: w187 -> [w190]
          tunnel: [w189] -> w185
          tunnel: w183 -> [w188]
          tunnel: w185 -> [w194]
          tunnel: [w194] -> w184
          tunnel: [w195] -> w186
          tunnel: w184 -> [w195]
          frame #0 {
            n217 = call-poly "Signals (Set).vi"("ISOBUS address"=w188, "PSU Act Stat"=T7 "HOLD", "Mercury Reference In"=w190) -> ("Mercury Reference Out"=w189:T4)  [unwired: 5 in, 3 out]
          }
          frame #1 {
            n218 = One Button Dialog(message="An error has been detected.\nThe current has been frozen where it is. Please look up the error code displayed\nand solve the issue to continue operation. To ramp down manually, press\n\"To Zero\" on the front panel of the Mercury iPS itself. ", button name ("OK")="OK") -> ()  [unwired: 1 out]
          }
          frame #2 {
            n219 = Stop() -> ()  [unwired: 1 in]
          }
        }
      }
    }
    n220 = call-poly "Signals (Read).vi"("ISOBUS address"=w65, "error in"=w102, "Mercury Reference In"=w103) -> ("error out"=w92:errorcluster, "PSU Act Stat"=w55:T7, "Mercury Reference Out"=w93:T4)  [unwired: 5 in, 1 out]
    n221 = case shown="True" w109 {
      tunnel: w72 -> [_ w181]
      tunnel: w46 -> [_ w167]
      tunnel: w56 -> [_ w163]
      tunnel: w55 -> [_ w161]
      frame False {
      }
      frame True {
        w162 = "\t"
        w164 = "A"
        n222 = Format Into String(w167) -> (resulting string=w166:string)  [unwired: 3 in, 1 out]
        n223 = Get Date/Time String(want seconds? (F)=TRUE) -> (date string=w173:string, time string=w171:string)  [unwired: 2 in]
        n224 = Format Into String(w181) -> (resulting string=w169:string)  [unwired: 3 in, 1 out]
        n225 = call <vilib>:"Space Constant.vi"() -> ("String"=w165:string)
        n226 = Open/Create/Replace File(file path (use dialog)=path "C:/Users/ptgroup/Downloads/ipsControl2013 new Folder/ipsControl2013 new Folder/C/Users/poltarg/Documents/lastcurrent.txt" ("file (use dialog)")) -> (refnum out=w179:refnum<file>)  [unwired: 5 in, 2 out]
        n227 = call <vilib>:"Space Constant.vi"() -> ("String"=w172:string)
        n228 = Get File Size(file=w179) -> (refnum out=w178:refnum<file>, size (in bytes)=w175:i64)  [unwired: 1 in, 1 out]
        n229 = Concatenate Strings(w173, w172, w171, "\t", w169, w165, w164, w162, w166, w165, w164, w162, w163, w162, w161, "\r\n") -> (w174:string)
        n230 = Set File Position(offset (in bytes) (0)=w175, refnum=w178) -> (refnum out=w177:refnum<file>)  [unwired: 2 in, 1 out]
        n231 = Write to Text File(file (use dialog)=w177, text=w174) -> (refnum out=w176:refnum<file>)  [unwired: 2 in, 2 out]
        n232 = Close File(refnum=w176) -> ()  [unwired: 1 in, 2 out]
      }
    }
    n233 = case shown="\"RTOS\"" w55 {
      tunnel: [TRUE FALSE FALSE TRUE] -> w101
      tunnel: [FALSE TRUE FALSE FALSE] -> w98
      tunnel: [FALSE FALSE TRUE FALSE] -> w99
      tunnel: [FALSE ("Blinking") FALSE ("Blinking") FALSE ("Blinking") TRUE ("Blinking")] -> w100
      tunnel: [TRUE FALSE FALSE TRUE] -> w68
      frame "HOLD", Default {
      }
      frame "RTOS" {
      }
      frame "RTOZ" {
      }
      frame "CLMP" {
      }
    }
    "Holdlight" <- w101
    "Setlight" <- w98
    "Zerolight" <- w99
    n234 = And(x=w68, y=w69) -> (x .and. y?=w67:bool)
    n235 = feedback-in #1(w67) -> ()
    n236 = property on="Holdlight" class="Bool (strict)"("Blinking"=w100) -> ()  [unwired: 2 in, 2 out]
    n237 = call-poly "Signals (Read).vi"("ISOBUS address"=w65, "error in"=w92, "Mercury Reference In"=w93) -> ("error out"=w88:errorcluster, "Level"=w91:dbl, "Mercury Reference Out"=w87:T4)  [unwired: 4 in, 2 out]
    "Helium Fill Level" <- w91
    n238 = Format Into String(w91) -> (resulting string=w78:string)  [unwired: 3 in, 1 out]
    n239 = call-poly "Signals (Read).vi"("ISOBUS address"=w65, "error in"=w88, "Mercury Reference In"=w87) -> ("error out"=w85:errorcluster, "Level"=w84:dbl, "Mercury Reference Out"=w86:T4)  [unwired: 4 in, 2 out]
    "Nitrogen Fill Level" <- w84
    n240 = Format Into String(w84) -> (resulting string=w73:string)  [unwired: 3 in, 1 out]
    n241 = String Subset(string=w73, length (rest)=5 ("length (rest)")) -> (substring=w74:string)  [unwired: 1 in]
    n242 = Concatenate Strings(w74, "%") -> (→"concatenated string 2":string)
    n243 = String Subset(string=w78, length (rest)=5 ("length (rest)")) -> (substring=w76:string)  [unwired: 1 in]
    n244 = Concatenate Strings(w76, "%") -> (→"concatenated string":string)
    "String" <- "SWITCH HEATER CHANGING STATE, PLEASE WAIT" ("String")
    "Baselinetext" <- "BASELINE MODE" ("Baselinetext")
    "Shim1Light" <- "Shim 1"
    "Shim2Light" <- "Shim 2"
  }
  n245 = call "close_relay.vi"("Handle"=w1) -> ()  [unwired: 9 in, 2 out]
  n246 = call "Close.vi"("error in (no error)"=w16, "Mercury Reference"=w17) -> ("error out"=w18:errorcluster)  [unwired: 9 in]
  n247 = global write "Global 2.vi" "Error Out"(w18) -> ()
